vi "Main Page.vi"(8 "error in (no error)":errorcluster, 11 "Node Ptr":T2 format="%.0x") -> (0 "error out":errorcluster)   [LabVIEW 2020, in "SLSC-12201 DIO System Explorer.lvlib"]
uses:
  SLSC-12201 DIO System Explorer.lvlib
  <vilib>/NI VeriStand/Custom Device API/Custom Device Item Ref.ctl
  Direction Control.ctl
  Shared/Constants.vi
  <vilib>/NI VeriStand/Custom Device Tools/Custom Device Utility Library/NI VeriStand - Search for All Items by Name.vi
  <vilib>/NI VeriStand/Custom Device API/Get Item Property (Boolean).vi
  <vilib>/NI VeriStand/Custom Device Tools/Custom Device Utility Library/NI VeriStand - Search for Item by Name.vi
  <vilib>/NI VeriStand/Custom Device API/Get Item Property (I32).vi
  <vilib>/NI VeriStand/Custom Device API/Get Item Property (Variant).vi
  <vilib>/NI VeriStand/Custom Device API/Set Item Property (Variant).vi
  SLSC Pinout Window.vi
  SLSC Diagram Window.vi
  <vilib>/NI VeriStand/Custom Device API/Set Item Property (Boolean).vi
  <vilib>/NI VeriStand/Custom Device API/Set Item Property (String).vi
  <vilib>/NI VeriStand/Custom Device API/Custom Device API.lvlib
  Shared/SLSC-12201 DIO Shared.lvlib
  <vilib>/NI VeriStand/Custom Device Tools/Custom Device Utility Library/Custom Device Utility Library.lvlib
panel:
  in  "Loop rate":u32
  in  "rev A":bool
  in  "SHDocVw.IWebBrowser2":refnum<k7>(container)
  out "Version":string
  in  "Direction":T1 items=["Input", "Output Source", "Output Sink", "Output Push-Pull"]
  in  "Apply":bool
  in  "Enable":bool
  in  "Disable":bool
  in  "Tab Control":enum32{"Bank 0", "Bank 1"}(tab)
  in  "Input Threshold 5V Bank 0":dbl caption="Input Threshold"
  in  "Bank0 Select Vsup":u16(ring) caption="Voltage Supply" items=["Off", "Vsup_0", "Vsup_1"]
  in  "Pullup Resistor Bank 0":bool
  in  "Input Threshold 33V Bank 0":dbl caption="Input Threshold"
  in  "Enable 5V Range Bank 0":bool
  in  "Input Threshold 5V Bank 1":dbl caption="Input Threshold"
  in  "Bank1 Select Vsup":u16(ring) caption="Voltage Supply" items=["Off", "Vsup_0", "Vsup_1"]
  in  "Enable 5V Range Bank 1":bool
  in  "Pullup Resistor Bank 1":bool
  in  "Input Threshold 33V Bank 1":dbl caption="Input Threshold"
  in  "Tree":string[](tree)
  in  "Make Static Only":bool
  in  "Title":cluster{"Section Name":string}={"Section Name"="Custom Device Properties"}
  out "Module Number":i32
  in  "Header":cluster{"Section Name":string}={"Section Name"="Custom Device Item Settings"}
  in  "Description":string
  in  "Name":string
  # "ms"
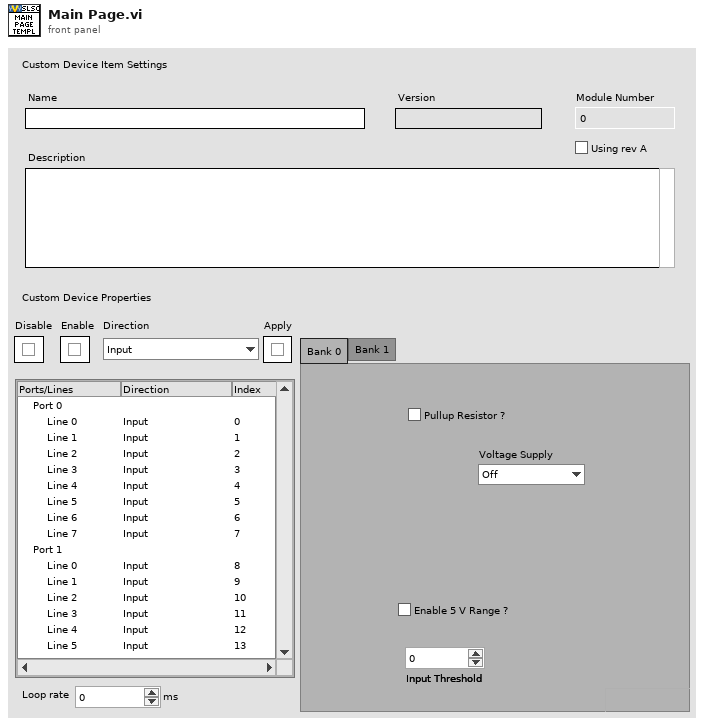
[diagram p1: front panel]
types:
  T1 = typedef "SLSC-12201 DIO System Explorer.lvlib/Direction Control.ctl" = u16
  T2 = typedef "Custom Device API.lvlib/Custom Device Item Ref.ctl" = u64
  T3 = enum8{"Enabled", "Disabled", "Disabled and Grayed Out"}
  T4 = typedef "Custom Device API.lvlib/Custom Device Channel.ctl" = cluster{"Type":T5, "Units":string, "Default Value":dbl, "Faultable":bool, "Scalable":bool}
  T5 = typedef "Custom Device API.lvlib/Custom Device Channel Type.ctl" = enum16{"Input", "Output"}
  T6 = cluster{"Channel Name":string, "SLSC Name":string, "Channel":T4, "Enum Names":string[], "Enum Values":i32[]}[]
  T7 = typedef "SLSC-12201 DIO System Explorer.lvlib/SLSC Channel Information.ctl" = cluster{"Channel Name":string, "SLSC Name":string, "Configuration":T4, "Enum Names":string[], "Enum Values":i32[]}
  T8 = typedef "Custom Device API.lvlib/Custom Device Item Info.ctl" = cluster{"Name":string, "Is Channel":bool, "GUID":string, "Is Waveform":bool}
  T9 = typedef "Custom Device API.lvlib/Custom Device Commands.ctl" = enum16{"Default", "Item renamed", "Shutdown", "Dynamic button pressed"}
  T10 = typedef "LVPoint32TypeDef.ctl" = cluster{"Horizontal":i32, "Vertical":i32}
  T11 = cluster{"Channel Name":string, "SLSC Name":string, "Channel":T4}[]
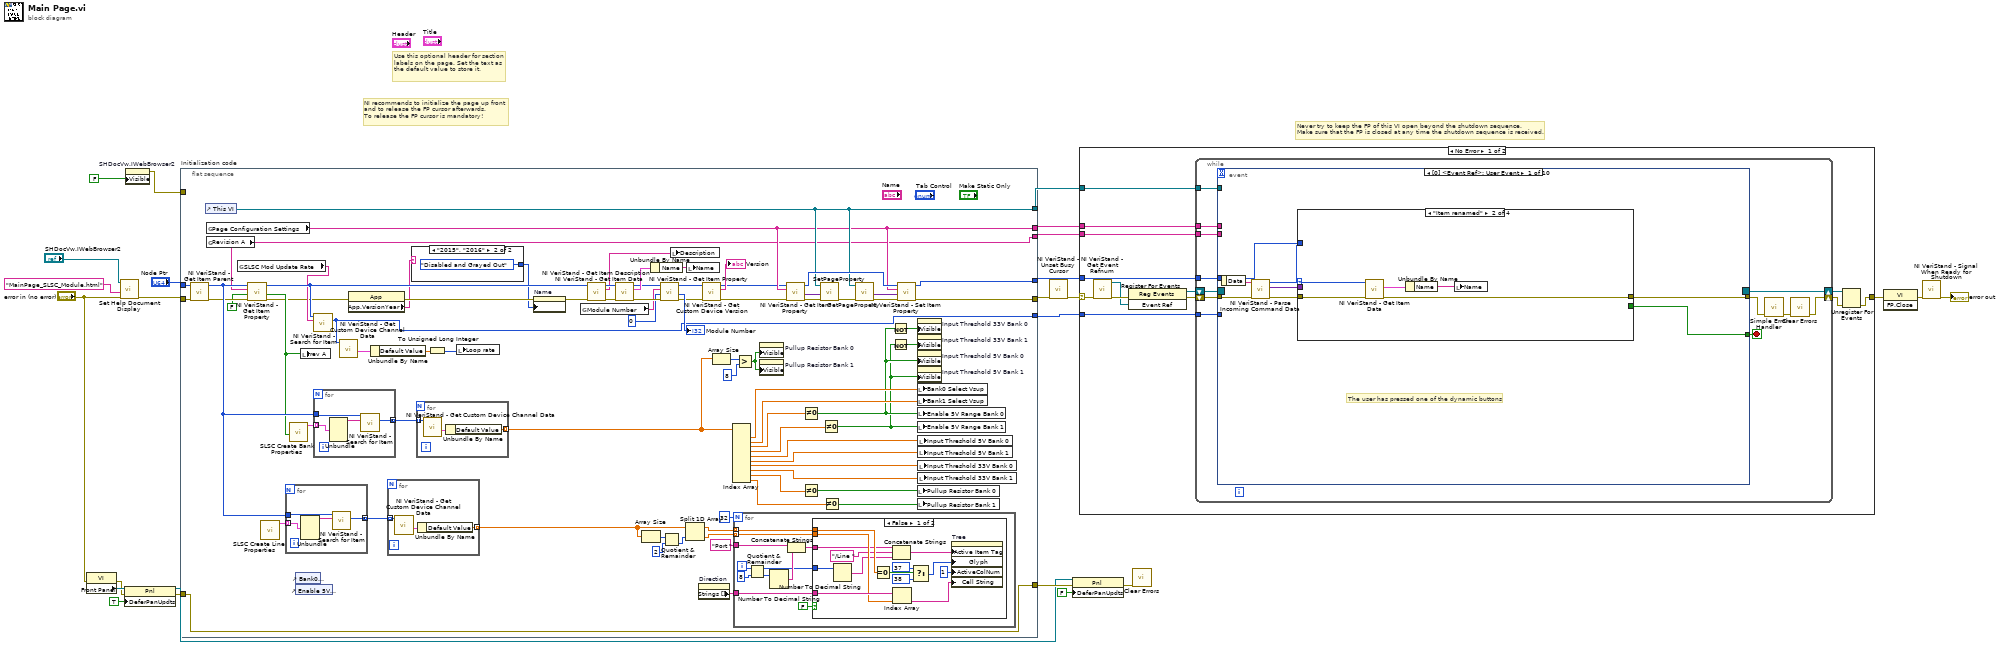
[diagram p0: block diagram]
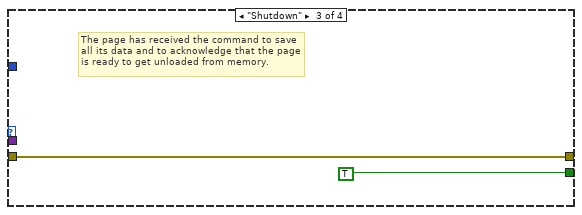
[diagram p3: hidden frame]
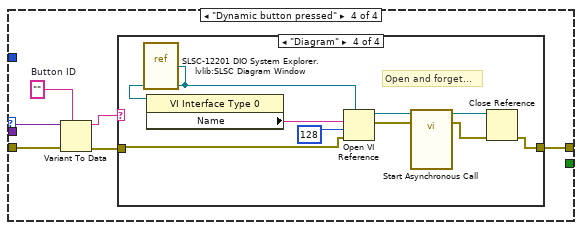
[diagram p4: hidden frame]
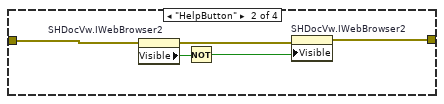
[diagram p6: hidden frame]
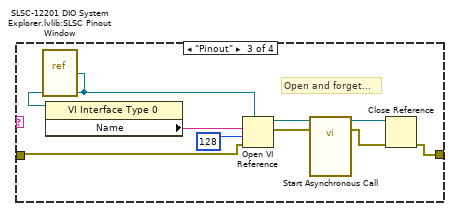
[diagram p7: hidden frame]
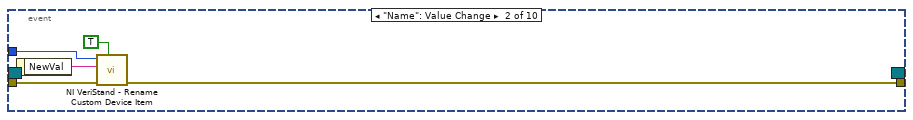
[diagram p8: hidden frame]
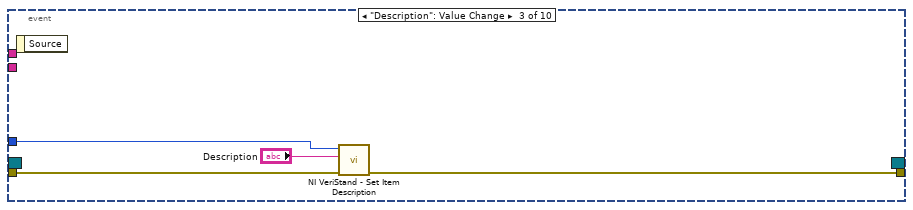
[diagram p9: hidden frame]
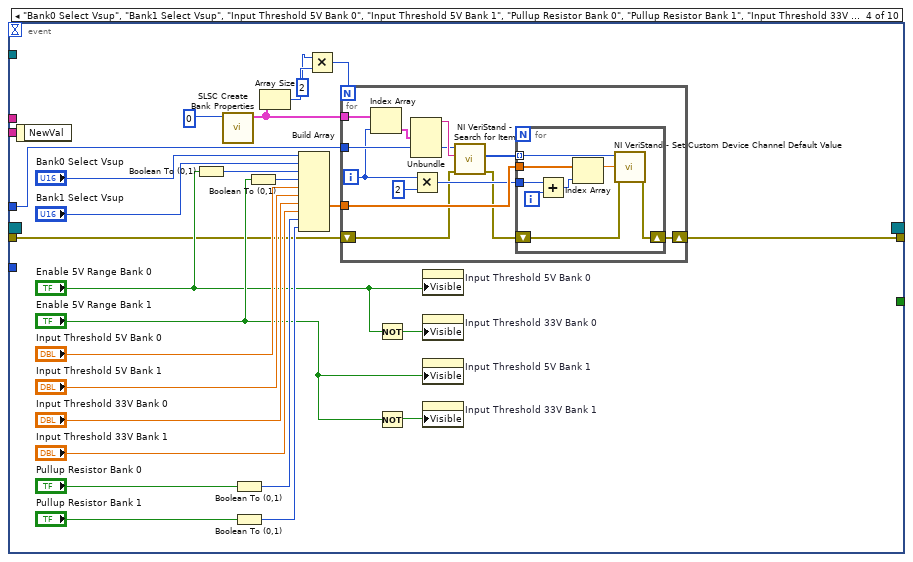
[diagram p10: hidden frame]
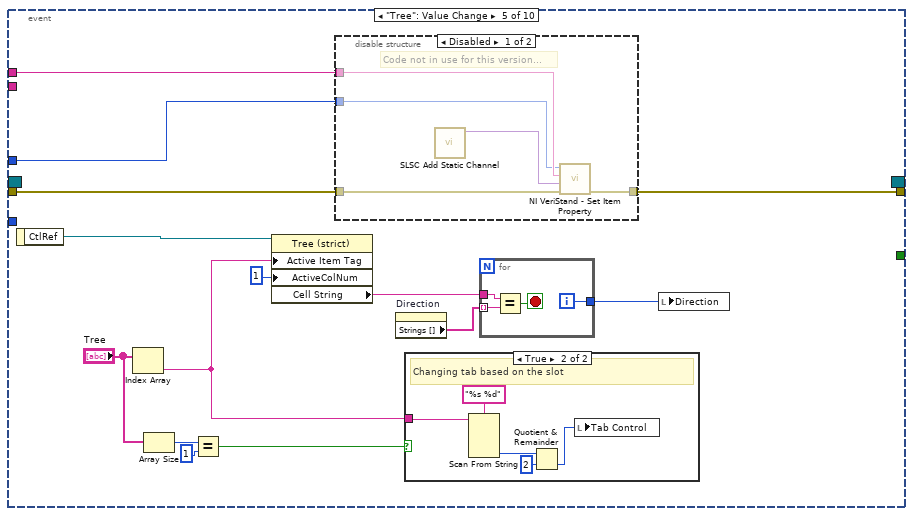
[diagram p11: hidden frame]
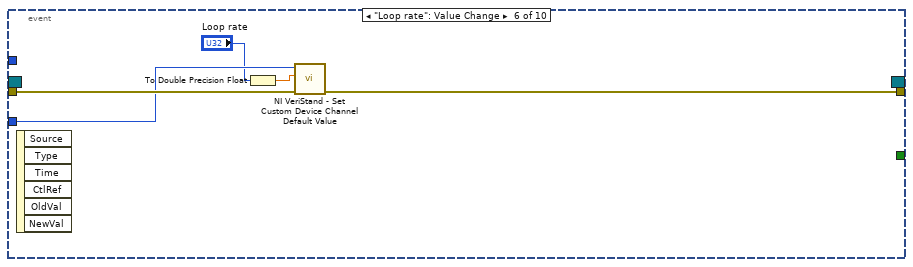
[diagram p14: hidden frame]
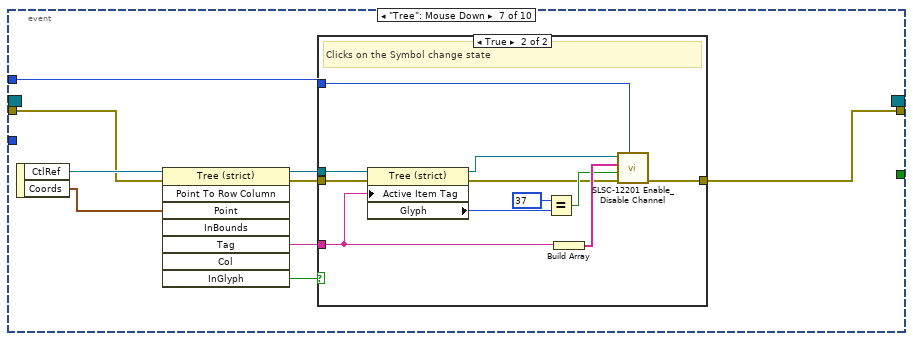
[diagram p15: hidden frame]
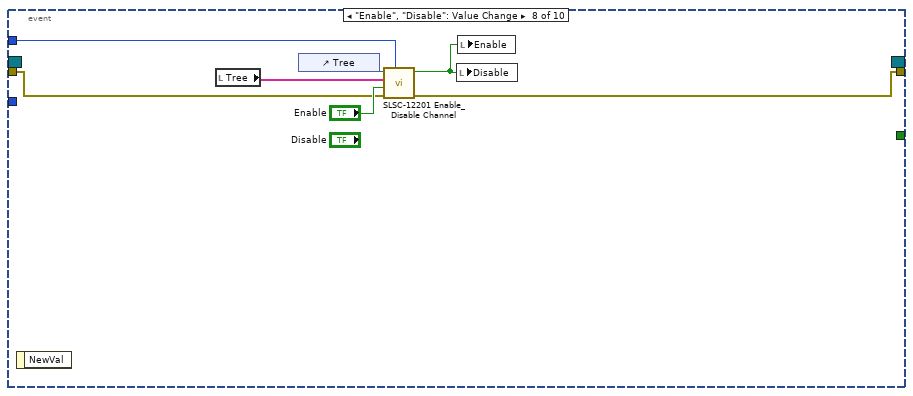
[diagram p17: hidden frame]
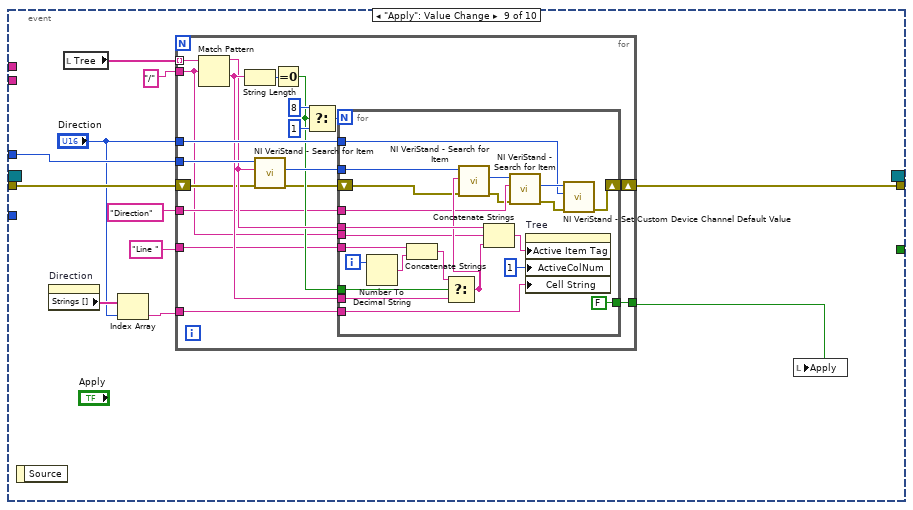
[diagram p18: hidden frame]
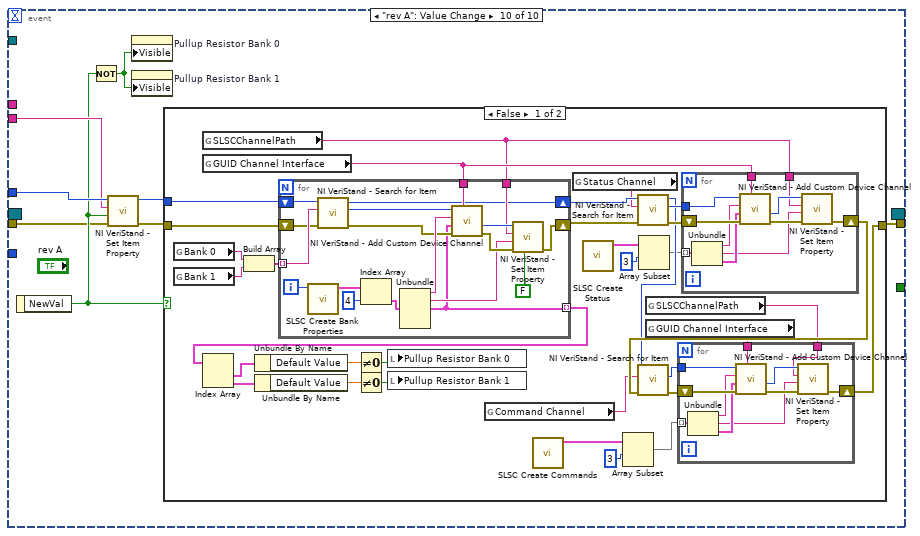
[diagram p19: hidden frame]
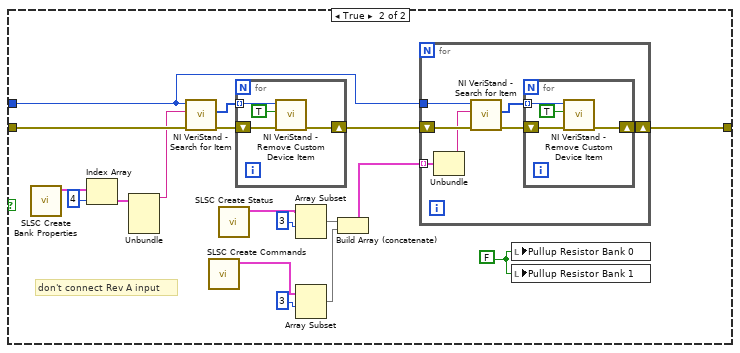
[diagram p20: hidden frame]
diagram:
  # "Never try to keep the FP of this VI open beyond the shutdown sequence.\nMake sure that the FP is closed at any time the shutdown sequence is received."
  # "Use this optional header for section labels on the page. Set the text as the default value to store it."
  # "NI recommends to initialize the page up front\nand to release the FP cursor afterwards.\nTo release the FP cursor is mandatory!"
  n1 = property class="VI"(error in="error in (no error)") -> (error out=w8:errorcluster, "Front Panel"=w10:refnum<vi>)  [unwired: 1 in, 1 out]
  n2 = call "Set Help Document Display.vi"("error in (no error)"="error in (no error)", "HTML File to Load"="MainPage_SLSC_Module.html" ("HTML File"), "SHDocVw.IWebBrowser2"="SHDocVw.IWebBrowser2") -> ("error out"=w13:errorcluster)  [unwired: 8 in]
  n3 = property class="Pnl"(reference=w10, error in=w8, "DeferPanUpdts"=TRUE ("Defer Panel Updates")) -> (reference out=w2:refnum<vi>, error out=w6:errorcluster)
  n4 = property on="SHDocVw.IWebBrowser2" class="AXCont"("Visible"=FALSE) -> (error out=w16:errorcluster)  [unwired: 2 in, 1 out]
  n5 = flat-sequence "Initialization code" {
    tunnel: w13 -> [w80]
    tunnel: "Node Ptr" -> [w81]
    tunnel: [w87] -> w21
    tunnel: [w84] -> w19
    tunnel: [w83] -> w18
    tunnel: [w82] -> w17
    tunnel: w16 -> [_]
    tunnel: [w38] -> w15
    tunnel: w6 -> [w36]
    tunnel: [w36] -> w4
    tunnel: [w30] -> w1
    frame #0 {
      n6 = call <vilib>:"NI VeriStand - Get Item Parent.vi"("error in (no error)"=w80, "Item Ref in"=w81) -> ("error out"=w40:errorcluster, "Item Ref out"=w41:T2)  [unwired: 6 in, 2 out]
      n7 = control-ref of="This VI"() -> (w83:refnum<vi>)
      n8 = global read "Constants.vi" "Page Configuration Settings"() -> (w82:string)
      n9 = global read "Constants.vi" "Revision A"() -> (w38:string)
      n10 = global read "Constants.vi" "SLSC Mod Update Rate"() -> (w31:string)
      n11 = call-poly <vilib>:"NI VeriStand - Get Item Property.vi"("error in (no error)"=w40, "Default Value"=FALSE, "Property Name"=w38, "Item Ref in"=w41) -> ("error out"=w29:errorcluster, "Value"=w37:bool, "Item Ref out"=w35:T2)  [unwired: 4 in, 1 out]
      n12 = call "SLSC Create Line Properties.vi"() -> ("Outgoing configuration"=w69:T6)  [unwired: 11 in]
      n13 = for {
        tunnel: w41 -> [w136]
        tunnel: w69 -> [w135] mode=indexing
        tunnel: [w134] -> w68 mode=concatenating
        n14 = Unbundle(w135) -> ("Channel Name"=w133:string)  [unwired: 4 out]
        n15 = call-poly <vilib>:"NI VeriStand - Search for Item.vi"("Item Name"=w133, "Section Ref in"=w136) -> ("Item Refs"=w134:T2[])  [unwired: 6 in, 3 out]
      }
      n16 = call "SLSC Create Bank Properties.vi"("RevA?"=w37) -> ("Outgoing configuration"=w76:T7[])  [unwired: 9 in, 1 out]
      n17 = control-ref of="Bank0 Select Vsup"() -> ()  [unwired: 1 out]
      n18 = control-ref of="Enable 5V Range Bank 0"() -> ()  [unwired: 1 out]
      n19 = local write "rev A"(w37) -> ()
      n20 = call-poly <vilib>:"NI VeriStand - Search for Item.vi"("Item Name"=w31, "Section Ref in"=w35) -> ("Item Ref"=w30:T2)  [unwired: 6 in, 3 out]
      n21 = for {
        tunnel: w41 -> [w140]
        tunnel: w76 -> [w138] mode=indexing
        tunnel: [w137] -> w75 mode=concatenating
        n22 = Unbundle(w138) -> ("Channel Name"=w139:string)  [unwired: 4 out]
        n23 = call-poly <vilib>:"NI VeriStand - Search for Item.vi"("Item Name"=w139, "Section Ref in"=w140) -> ("Item Refs"=w137:T2[])  [unwired: 6 in, 3 out]
      }
      n24 = call <vilib>:"NI VeriStand - Get Custom Device Channel Data.vi"("Channel Ref in"=w30) -> ("Channel"=w34:T4)  [unwired: 5 in, 5 out]
      n25 = property class="App"(error in=w29) -> (error out=w28:errorcluster, "App.VersionYear"=w27:string)  [unwired: 1 in, 1 out]
      n26 = Unbundle By Name(w34) -> ("Default Value"=w33:dbl)
      n27 = for {
        tunnel: [w132] -> w62 mode=indexing
        tunnel: w68 -> [w131] mode=indexing
        n28 = call <vilib>:"NI VeriStand - Get Custom Device Channel Data.vi"("Channel Ref in"=w131) -> ("Channel"=w130:T4)  [unwired: 5 in, 5 out]
        n29 = Unbundle By Name(w130) -> ("Default Value"=w132:dbl)
      }
      n30 = case shown="\"2015\", \"2016\"" w27 {
        tunnel: [T3."Enabled" ("Disabled") T3."Disabled and Grayed Out" ("Disabled")] -> w26
        frame "False", Default {
        }
        frame "2015", "2016" {
        }
      }
      n31 = for {
        tunnel: [w143] -> w54 mode=indexing
        tunnel: w75 -> [w142] mode=indexing
        n32 = call <vilib>:"NI VeriStand - Get Custom Device Channel Data.vi"("Channel Ref in"=w142) -> ("Channel"=w141:T4)  [unwired: 5 in, 5 out]
        n33 = Unbundle By Name(w141) -> ("Default Value"=w143:dbl)
      }
      n34 = To Unsigned Long Integer(number=w33) -> (unsigned 32bit integer=w32:u32)
      n35 = local write "Loop rate"(w32) -> ()
      n36 = property on="Name" class="Str"(error in=w28, "DisabledEnum"=w26) -> (error out=w97:errorcluster)  [unwired: 1 in, 1 out]
      n37 = global read "Constants.vi" "Module Number"() -> (w94:string)
      n38 = call <vilib>:"NI VeriStand - Get Item Description.vi"("error in (no error)"=w97, "Item Ref in"=w35) -> ("error out"=w100:errorcluster, "Description"=w101:string, "Item Ref out"=w102:T2)  [unwired: 7 out]
      n39 = call <vilib>:"NI VeriStand - Get Item Data.vi"("error in (no error)"=w100, "Item Ref in"=w102) -> ("error out"=w95:errorcluster, "Item Info"=w99:T8, "Item Ref out"=w93:T2)  [unwired: 7 out]
      n40 = Array Size(array=w62) -> (size(s)=w61:i32)
      n41 = Unbundle By Name(w99) -> ("Name"=w98:string)
      n42 = call-poly <vilib>:"NI VeriStand - Get Item Property.vi"("error in (no error)"=w95, "Default Value"=0, "Property Name"=w94, "Item Ref in"=w93) -> ("error out"=w45:errorcluster, "Value"=→"Module Number":i32, "Item Ref out"=w43:T2)  [unwired: 4 in, 1 out]
      n43 = Quotient & Remainder(x=w61, y=2) -> (floor(x/y)=w59:i32)  [unwired: 1 out]
      n44 = local write "Description"(w101) -> ()
      n45 = Split 1D Array(array=w62, index=w59) -> (first subarray=w67:dbl[], second subarray=w66:dbl[])
      n46 = local write "Name"(w98) -> ()
      n47 = property on="Direction" class="Ring (strict)"() -> ("Strings []"=w65:string[])  [unwired: 2 in, 2 out]
      n48 = call <vilib>:"NI VeriStand - Get Custom Device Version.vi"("error in (no error)"=w45, "Device Ref in"=w43) -> ("error out"=w44:errorcluster, "Value"=→"Version":string, "Device Ref out"=w42:T2)  [unwired: 7 in]
      n49 = Array Size(array=w54) -> (size(s)=w53:i32)
      n50 = Index Array(array=w54) -> (element #1=w79:dbl, element #2=w74:dbl, element #3=w73:dbl, element #4=w72:dbl, element #5=w58:dbl, element #6=w57:dbl, element #7=w56:dbl, element #8=w55:dbl, element #9=w71:dbl, element #10=w70:dbl)  [unwired: 10 in]
      n51 = for {
        N: 32 -> [_]
        tunnel: w67 -> [w115] mode=indexing
        tunnel: w66 -> [w113] mode=indexing
        tunnel: w65 -> [w114]
        tunnel: "Port " ("y") -> [w109]
        i -> [w112]
        n52 = Quotient & Remainder(x=w112, y=8) -> (x-y*floor(x/y)=w106:i32, floor(x/y)=w110:i32)
        n53 = Number To Decimal String(number=w110) -> (decimal integer string=w108:string)  [unwired: 1 in]
        n54 = Concatenate Strings(w109, w108) -> (w107:string)
        n55 = case shown="False" FALSE {
          tunnel: w115 -> [w125 _]
          tunnel: w114 -> [w123 _]
          tunnel: w113 -> [w122 _]
          tunnel: w107 -> [w118 _]
          tunnel: w106 -> [w116 _]
          frame False {
            n56 = Number To Decimal String(number=w116) -> (decimal integer string=w119:string)  [unwired: 1 in]
            n57 = Equal To 0?(x=w125) -> (x = 0?=w127:bool)
            n58 = Concatenate Strings(w118, "/Line " ("string"), w119) -> (w117:string)
            n59 = Index Array(array=w123, index=w122) -> (element=w121:string)
            n60 = Select(t=37, s=w127, f=38) -> (s? t:f=w126:i32)
            n61 = property on="Tree" class="Tree (strict)"("Active Item Tag"=w117, "Glyph"=w126, "ActiveColNum"=1 ("Active Cell:Active Column Number"), "Cell String"=w121) -> ()  [unwired: 2 in, 2 out]
          }
          frame True {
          }
        }
      }
      n62 = Greater?(x=w53, y=8) -> (0:w47:bool)
      n63 = property on="Pullup Resistor Bank 0" class="Bool (strict)"("Visible"=w47) -> ()  [unwired: 2 in, 2 out]
      n64 = property on="Pullup Resistor Bank 1" class="Bool (strict)"("Visible"=w47) -> ()  [unwired: 2 in, 2 out]
      n65 = call-poly <vilib>:"NI VeriStand - Get Item Property.vi"("error in (no error)"=w44, "Property Name"=w82, "Item Ref in"=w42) -> ("error out"=w91:errorcluster, "Value"=w90:variant, "Item Ref out"=w86:T2)  [unwired: 5 in, 1 out]
      n66 = Not Equal To 0?(x=w73) -> (x != 0?=w49:bool)
      n67 = Not Equal To 0?(x=w71) -> (x != 0?=w78:bool)
      n68 = call "SetPageProperty.vi"("error in"=w91, "variant"=w90, "This VI"=w83) -> ("error out"=w89:errorcluster)  [unwired: 8 in]
      n69 = Not Equal To 0?(x=w72) -> (x != 0?=w48:bool)
      n70 = Not Equal To 0?(x=w70) -> (x != 0?=w77:bool)
      n71 = call "GetPageProperty.vi"("error in (no error)"=w89, "This VI"=w83) -> ("error out"=w88:errorcluster, "Settings"=w85:variant)  [unwired: 8 in]
      n72 = Not(x=w49) -> (.not. x?=w51:bool)
      n73 = Not(x=w48) -> (.not. x?=w50:bool)
      n74 = call-poly <vilib>:"NI VeriStand - Set Item Property.vi"("error in (no error)"=w88, "Value"=w85, "Property Name"=w82, "Item Ref in"=w86) -> ("error out"=w87:errorcluster, "Item Ref out"=w84:T2)  [unwired: 5 in, 1 out]
      n75 = property on="Input Threshold 33V Bank 0" class="DigNum (strict)"("Visible"=w51) -> ()  [unwired: 2 in, 2 out]
      n76 = property on="Input Threshold 33V Bank 1" class="DigNum (strict)"("Visible"=w50) -> ()  [unwired: 2 in, 2 out]
      n77 = property on="Input Threshold 5V Bank 0" class="DigNum (strict)"("Visible"=w49) -> ()  [unwired: 2 in, 2 out]
      n78 = property on="Input Threshold 5V Bank 1" class="DigNum (strict)"("Visible"=w48) -> ()  [unwired: 2 in, 2 out]
      n79 = local write "Bank0 Select Vsup"(w79) -> ()
      n80 = local write "Bank1 Select Vsup"(w74) -> ()
      n81 = local write "Enable 5V Range Bank 0"(w49) -> ()
      n82 = local write "Enable 5V Range Bank 1"(w48) -> ()
      n83 = local write "Pullup Resistor Bank 0"(w78) -> ()
      n84 = local write "Pullup Resistor Bank 1"(w77) -> ()
      n85 = local write "Input Threshold 5V Bank 0"(w58) -> ()
      n86 = local write "Input Threshold 5V Bank 1"(w57) -> ()
      n87 = local write "Input Threshold 33V Bank 0"(w56) -> ()
      n88 = local write "Input Threshold 33V Bank 1"(w55) -> ()
    }
  }
  n89 = call <vilib>:"NI VeriStand - Unset Busy Cursor.vi"("error in (no error)"=w21) -> ("error out"=w20:errorcluster)  [unwired: 10 out]
  n90 = property class="Pnl"(reference=w2, error in=w4, "DeferPanUpdts"=FALSE ("Defer Panel Updates")) -> (error out=w3:errorcluster)  [unwired: 1 out]
  n91 = case shown="No Error" w20 {
    selector: w20 -> [w148 w500]
    tunnel: [w153 w498] -> w25
    tunnel: w19 -> [w149 _]
    tunnel: w18 -> [w147 _]
    tunnel: w17 -> [w146 _]
    tunnel: w15 -> [w145 _]
    tunnel: w1 -> [w144 _]
    frame No Error {
      n92 = call <vilib>:"NI VeriStand - Get Event Refnum.vi"("error in (no error)"=w148) -> ("error out"=w156:errorcluster, "Event Ref"=w152:refnum<user-event>)  [unwired: 9 out]
      n93 = register-events(error in=w156, w152) -> (reference out=w150:refnum<event-registration>, error out=w151:errorcluster)  [unwired: 1 in]
      n94 = while {
        tunnel: w149 -> [w164]
        shift-right: [w161] -> w154
        shift-left: w151 -> [w167]
        shift-right: [w168] -> w155
        shift-left: w150 -> [w166]
        tunnel: w147 -> [w160]
        tunnel: w146 -> [w159]
        tunnel: w145 -> [w158]
        tunnel: w144 -> [w157]
        stop <- w165 stop-if-true
        n95 = event shown="[0] <Event Ref>: User Event" {
          selector: w166 -> [_ _ _ _ _ _ _ _ _ _]
          dyn-events: [_ _ _ _ _ _ _ _ _ _] -> w168
          timeout: _ -> [_ _ _ _ _ _ _ _ _ _]
          tunnel: w167 -> [w176 w218 w222 w225 w281 w301 w309 w326 w335 w384]
          tunnel: [w172 _ _ _ _ _ _ _ _ _] -> w165
          tunnel: [w171 w217 w221 w224 w282 w300 w305 w325 w334 w390] -> w163
          tunnel: w164 -> [w170 w219 w223 w247 w279 _ w306 w329 w340 w388]
          tunnel: w160 -> [_ _ _ _ _ _ _ _ _ _]
          tunnel: w159 -> [_ _ _ _ w280 _ _ _ _ _]
          tunnel: w158 -> [_ _ _ _ _ _ _ _ _ w386]
          tunnel: w157 -> [_ _ _ _ _ w299 _ _ _ _]
          event User Event {
            # "The user has pressed one of the dynamic buttons"
            n96 = event-data() -> ("Data"=w175:string)  [unwired: 1 out]
            n97 = call <vilib>:"NI VeriStand - Parse Incoming Command Data.vi"("error in (no error)"=w176, "Incoming data"=w175) -> ("error out"=w174:errorcluster, "Outgoing data"=w169:variant, "Action"=w173:T9)  [unwired: 7 out]
            n98 = case shown="\"Item renamed\"" w173 {
              tunnel: w174 -> [w177 w182 w183 w190]
              tunnel: [_ _ TRUE _] -> w172
              tunnel: [w177 w179 w183 w185] -> w171
              tunnel: w170 -> [_ w181 _ _]
              tunnel: w169 -> [_ _ _ w189]
              frame "Default", Default {
              }
              frame "Item renamed" {
                n99 = call <vilib>:"NI VeriStand - Get Item Data.vi"("error in (no error)"=w182, "Item Ref in"=w181) -> ("error out"=w179:errorcluster, "Item Info"=w180:T8)  [unwired: 8 out]
                n100 = Unbundle By Name(w180) -> ("Name"=w178:string)
                n101 = local write "Name"(w178) -> ()
              }
              frame "Shutdown" {
                # "The page has received the command to save all its data and to acknowledge that the page is ready to get unloaded from memory."
              }
              frame "Dynamic button pressed" {
                w188 = ""  # Button ID
                n102 = Variant To Data(error in=w190, type=w188, Variant=w189) -> (data=w187:string, error out=w186:errorcluster)
                n103 = case shown="\"Diagram\"" w187 {
                  tunnel: w186 -> [w191 w194 w198 w207]
                  tunnel: [w191 w192 w199 w208] -> w185
                  frame Default {
                  }
                  frame "HelpButton" {
                    n104 = property on="SHDocVw.IWebBrowser2" class="AXCont"(error in=w194) -> (error out=w193:errorcluster, "Visible"=w196:bool)  [unwired: 1 in, 1 out]
                    n105 = Not(x=w196) -> (.not. x?=w195:bool)
                    n106 = property on="SHDocVw.IWebBrowser2" class="AXCont"(error in=w193, "Visible"=w195) -> (error out=w192:errorcluster)  [unwired: 1 in, 1 out]
                  }
                  frame "Pinout" {
                    # "Open and forget..."
                    n107 = vi-ref "SLSC-12201 DIO System Explorer.lvlib:SLSC Pinout Window.vi"() -> (w197:refnum<vi>)
                    n108 = property class="VI Interface Type 0"(reference=w197) -> ("Name"=w205:string)  [unwired: 1 in, 2 out]
                    n109 = Open VI Reference(type specifier VI Refnum (for type only)=w197, vi path=w205, options=128, error in (no error)=w198) -> (vi reference=w201:refnum<vi>, error out=w203:errorcluster)  [unwired: 2 in]
                    n110 = call-by-ref "Start Asynchronous Call"(reference=w201, error in=w203) -> (reference out=w202:refnum<vi>, error out=w204:errorcluster)  [unwired: 12 in]
                    n111 = Close Reference(reference=w202, error in (no error)=w204) -> (error out=w199:errorcluster)
                  }
                  frame "Diagram" {
                    # "Open and forget..."
                    n112 = vi-ref "SLSC-12201 DIO System Explorer.lvlib:SLSC Diagram Window.vi"() -> (w206:refnum<vi>)
                    n113 = property class="VI Interface Type 0"(reference=w206) -> ("Name"=w214:string)  [unwired: 1 in, 2 out]
                    n114 = Open VI Reference(type specifier VI Refnum (for type only)=w206, vi path=w214, options=128, error in (no error)=w207) -> (vi reference=w210:refnum<vi>, error out=w212:errorcluster)  [unwired: 2 in]
                    n115 = call-by-ref "Start Asynchronous Call"(reference=w210, error in=w212) -> (reference out=w211:refnum<vi>, error out=w213:errorcluster)  [unwired: 12 in]
                    n116 = Close Reference(reference=w211, error in (no error)=w213) -> (error out=w208:errorcluster)
                  }
                }
              }
            }
          }
          event "Name": Value Change {
            n117 = event-data() -> ("NewVal"=w216:string)  [unwired: 1 out]
            n118 = call <vilib>:"NI VeriStand - Rename Custom Device Item.vi"("Force Rename (F)"=TRUE, "error in (no error)"=w218, "New Name"=w216, "Item Ref in"=w219) -> ("error out"=w217:errorcluster)  [unwired: 7 out]
          }
          event "Description": Value Change {
            n119 = event-data() -> ()  [unwired: 2 out]
            n120 = call <vilib>:"NI VeriStand - Set Item Description.vi"("error in (no error)"=w222, "Description"="Description", "Item Ref in"=w223) -> ("error out"=w221:errorcluster)  [unwired: 8 out]
          }
          event "Bank0 Select Vsup", "Bank1 Select Vsup", "Input Threshold 5V Bank 0", "Input Threshold 5V Bank 1", "Pullup Resistor Bank 0", "Pullup Resistor Bank 1", "Input Threshold 33V Bank 0", "Input Threshold 33V Bank 1", "Enable 5V Range Bank 1", "Enable 5V Range Bank 0": Value Change {
            n121 = event-data() -> ()  [unwired: 2 out]
            n122 = Boolean To (0,1)(Boolean="Enable 5V Range Bank 0") -> (0, 1=w243:i16)
            n123 = call "SLSC Create Bank Properties.vi"("Bank Number"=0) -> ("Outgoing configuration"=w233:T7[])  [unwired: 9 in, 1 out]
            n124 = Boolean To (0,1)(Boolean="Pullup Resistor Bank 0") -> (0, 1=w235:i16)
            n125 = Boolean To (0,1)(Boolean="Pullup Resistor Bank 1") -> (0, 1=w234:i16)
            n126 = Boolean To (0,1)(Boolean="Enable 5V Range Bank 1") -> (0, 1=w242:i16)
            n127 = Array Size(array=w233) -> (size(s)=w231:i32)
            n128 = Build Array("Bank0 Select Vsup", "Bank1 Select Vsup", w243, w242, "Input Threshold 5V Bank 0", "Input Threshold 5V Bank 1", "Input Threshold 33V Bank 0", "Input Threshold 33V Bank 1", w235, w234) -> (w244:dbl[])
            n129 = Multiply(x=2 ("y"), y=w231) -> (x*y=w232:i32)
            n130 = for {
              N: w232 -> [_]
              tunnel: w247 -> [w259]
              tunnel: w244 -> [w257]
              tunnel: w233 -> [w256]
              shift-right: [w249] -> w224
              shift-left: w225 -> [w251]
              i -> [w253]
              n131 = Index Array(array=w256, index=w253) -> (element=w255:T7)
              n132 = Unbundle(w255) -> ("Channel Name"=w260:string)  [unwired: 4 out]
              n133 = Multiply(x=w253, y=2) -> (x*y=w252:i32)
              n134 = call-poly <vilib>:"NI VeriStand - Search for Item.vi"("error in"=w251, "Item Name"=w260, "Section Ref in"=w259) -> ("error out"=w250:errorcluster, "Item Refs"=w258:T2[])  [unwired: 5 in, 2 out]
              n135 = for {
                tunnel: w257 -> [w268]
                tunnel: w258 -> [w267] mode=indexing
                tunnel: w252 -> [w263]
                shift-right: [w261] -> w249
                shift-left: w250 -> [w262]
                i -> [w265]
                n136 = Add(x=w263, y=w265) -> (x+y=w264:i32)
                n137 = Index Array(array=w268, index=w264) -> (element=w266:dbl)
                n138 = call <vilib>:"NI VeriStand - Set Custom Device Channel Default Value.vi"("error in (no error)"=w262, "Default Value"=w266, "Channel Ref in"=w267) -> ("error out"=w261:errorcluster)  [unwired: 7 in, 1 out]
              }
            }
            n139 = Not(x="Enable 5V Range Bank 0") -> (.not. x?=w229:bool)
            n140 = Not(x="Enable 5V Range Bank 1") -> (.not. x?=w228:bool)
            n141 = property on="Input Threshold 5V Bank 0" class="DigNum (strict)"("Visible"="Enable 5V Range Bank 0") -> ()  [unwired: 2 in, 2 out]
            n142 = property on="Input Threshold 33V Bank 0" class="DigNum (strict)"("Visible"=w229) -> ()  [unwired: 2 in, 2 out]
            n143 = property on="Input Threshold 5V Bank 1" class="DigNum (strict)"("Visible"="Enable 5V Range Bank 1") -> ()  [unwired: 2 in, 2 out]
            n144 = property on="Input Threshold 33V Bank 1" class="DigNum (strict)"("Visible"=w228) -> ()  [unwired: 2 in, 2 out]
          }
          event "Tree": Value Change {
            n145 = event-data() -> ("CtlRef"=w278:refnum<vi>)  [unwired: 1 out]
            n146 = Index Array(array="Tree") -> (element=w269:string)  [unwired: 1 in]
            n147 = Array Size(array="Tree") -> (size(s)=w272:i32)
            n148 = Equal?(x=w272, y=1) -> (x = y?=w270:bool)
            n149 = property on="Property Node" class="Tree (strict)"(reference=w278, "Active Item Tag"=w269, "ActiveColNum"=1 ("Active Cell:Active Column Number")) -> ("Cell String"=w275:string)  [unwired: 1 in, 2 out]
            n150 = disable-structure shown="Disabled" {
              disable-tunnel: [w296 w297] -> w282
              disable-tunnel: w281 -> [w295 w297]
              disable-tunnel: w280 -> [w293 _]
              disable-tunnel: w279 -> [w292 _]
              frame Disabled {
                # "Code not in use for this version..."
                n151 = call "SLSC Add Static Channel.vi"() -> ("variant out"=w294:variant)  [unwired: 10 in, 1 out]
                n152 = call-poly <vilib>:"NI VeriStand - Set Item Property.vi"("error in (no error)"=w295, "Value"=w294, "Property Name"=w293, "Item Ref in"=w292) -> ("error out"=w296:errorcluster)  [unwired: 5 in, 2 out]
              }
              frame Enabled {
              }
            }
            n153 = property on="Direction" class="Ring (strict)"() -> ("Strings []"=w276:string[])  [unwired: 2 in, 2 out]
            n154 = case shown="True" w270 {
              tunnel: w269 -> [_ w286]
              frame False {
              }
              frame True {
                # "Changing tab based on the slot"
                n155 = Scan From String(format string="%s %d", input string=w286) -> (output 2=w285:i32)  [unwired: 5 in, 3 out]
                n156 = Quotient & Remainder(x=w285, y=2) -> (floor(x/y)=w283:i32)  [unwired: 1 out]
                n157 = local write "Tab Control"(w283) -> ()
              }
            }
            n158 = for {
              tunnel: w276 -> [w291] mode=indexing
              tunnel: w275 -> [w290]
              tunnel: [w288] -> w274
              i -> [w288]
              stop <- w289 stop-if-true
              n159 = Equal?(x=w290, y=w291) -> (x = y?=w289:bool)
            }
            n160 = local write "Direction"(w274) -> ()
          }
          event "Loop rate": Value Change {
            n161 = event-data() -> ()  [unwired: 7 out]
            n162 = To Double Precision Float(number="Loop rate") -> (double precision float=w302:dbl)
            n163 = call <vilib>:"NI VeriStand - Set Custom Device Channel Default Value.vi"("error in (no error)"=w301, "Default Value"=w302, "Channel Ref in"=w299) -> ("error out"=w300:errorcluster)  [unwired: 7 in, 1 out]
          }
          event "Tree": Mouse Down {
            n164 = event-data() -> ("CtlRef"=w311:refnum<vi>, "Coords"=w310:T10)  [unwired: 1 out]
            n165 = invoke class="Tree (strict)" method="Point To Row Column"(reference=w311, error in=w309, "Point"=w310) -> (reference out=w304:refnum<vi>, error out=w303:errorcluster, "Tag"=w307:string, "InGlyph"=w308:bool)  [unwired: 5 in, 4 out]
            n166 = case shown="True" w308 {
              tunnel: w307 -> [_ w318]
              tunnel: w306 -> [_ w322]
              tunnel: [w312 w321] -> w305
              tunnel: w304 -> [_ w320]
              tunnel: w303 -> [w312 w314]
              frame False {
              }
              frame True {
                # "Clicks on the Symbol change state"
                n167 = property on="Property Node" class="Tree (strict)"(reference=w320, error in=w314, "Active Item Tag"=w318) -> (reference out=w319:refnum<vi>, error out=w313:errorcluster, "Glyph"=w317:i32)
                n168 = Equal?(x=37, y=w317) -> (x = y?=w315:bool)
                n169 = Build Array(w318) -> (w323:string[])
                n170 = call "SLSC-12201 Enable_Disable Channel.vi"("Item Ref in"=w322, "error in (no error)"=w313, "Enable"=w315, "Tree"=w323, "TreeControl in"=w319) -> ("error out"=w321:errorcluster)  [unwired: 5 in, 1 out]
              }
            }
          }
          event "Enable", "Disable": Value Change {
            n171 = event-data() -> ()  [unwired: 2 out]
            n172 = local read "Tree"() -> (w330:string[])
            n173 = control-ref of="Tree"() -> (w324:refnum<vi>)
            n174 = call "SLSC-12201 Enable_Disable Channel.vi"("Item Ref in"=w329, "error in (no error)"=w326, "Enable"="Enable", "Tree"=w330, "TreeControl in"=w324) -> ("error out"=w325:errorcluster, "Boolean"=w327:bool)  [unwired: 5 in]
            n175 = local write "Disable"(w327) -> ()
            n176 = local write "Enable"(w327) -> ()
          }
          event "Apply": Value Change {
            n177 = event-data() -> ()  [unwired: 2 out]
            n178 = property on="Direction" class="Ring (strict)"() -> ("Strings []"=w333:string[])  [unwired: 2 in, 2 out]
            n179 = local read "Tree"() -> (w341:string[])
            n180 = Index Array(array=w333, index="Direction") -> (element=w331:string)
            n181 = for {
              tunnel: w341 -> [w354] mode=indexing
              tunnel: w331 -> [w356]
              tunnel: w340 -> [w355]
              tunnel: "Direction" -> [w352]
              tunnel: [w350] -> w339
              tunnel: "/" ("regular expression") -> [w342]
              tunnel: "Line " ("string") -> [w347]
              tunnel: "Direction" ("Item Name") -> [w346]
              shift-right: [w343] -> w334
              shift-left: w335 -> [w345]
              n182 = Match Pattern(string=w354, regular expression=w342) -> (before substring=w349:string, after substring=w351:string)  [unwired: 1 in, 2 out]
              n183 = String Length(string=w351) -> (length=w360:i32)
              n184 = call-poly <vilib>:"NI VeriStand - Search for Item.vi"("error in"=w345, "Item Name"=w349, "Section Ref in"=w355) -> ("error out"=w344:errorcluster, "Item Ref"=w353:T2)  [unwired: 5 in, 2 out]
              n185 = Equal To 0?(x=w360) -> (x = 0?=w348:bool)
              n186 = Select(t=8, s=w348, f=1) -> (s? t:f=w359:i32)
              n187 = for {
                N: w359 -> [_]
                tunnel: w349 -> [w379]
                tunnel: w356 -> [w361]
                tunnel: w353 -> [w380]
                tunnel: w352 -> [w362]
                tunnel: w348 -> [w376]
                tunnel: w351 -> [w373]
                tunnel: [FALSE] -> w350
                tunnel: w347 -> [w371]
                tunnel: w346 -> [w370]
                shift-right: [w366] -> w343
                shift-left: w344 -> [w369]
                tunnel: w342 -> [w365]
                i -> [w382]
                n188 = Number To Decimal String(number=w382) -> (decimal integer string=w381:string)  [unwired: 1 in]
                n189 = Concatenate Strings(w371, w381) -> (w375:string)
                n190 = Select(t=w375, s=w376, f=w373) -> (s? t:f=w374:string)
                n191 = call-poly <vilib>:"NI VeriStand - Search for Item.vi"("error in"=w369, "Item Name"=w374, "Section Ref in"=w380) -> ("error out"=w368:errorcluster, "Item Ref"=w378:T2)  [unwired: 5 in, 2 out]
                n192 = Concatenate Strings(w379, w365, w374) -> (w364:string)
                n193 = call-poly <vilib>:"NI VeriStand - Search for Item.vi"("error in"=w368, "Item Name"=w370, "Section Ref in"=w378) -> ("error out"=w367:errorcluster, "Item Ref"=w377:T2)  [unwired: 5 in, 2 out]
                n194 = property on="Tree" class="Tree (strict)"("Active Item Tag"=w364, "ActiveColNum"=1 ("Active Cell:Active Column Number"), "Cell String"=w361) -> ()  [unwired: 2 in, 2 out]
                n195 = call <vilib>:"NI VeriStand - Set Custom Device Channel Default Value.vi"("error in (no error)"=w367, "Default Value"=w362, "Channel Ref in"=w377) -> ("error out"=w366:errorcluster)  [unwired: 7 in, 1 out]
              }
            }
            n196 = local write "Apply"(w339) -> ()
          }
          event "rev A": Value Change {
            n197 = event-data() -> ("NewVal"=w385:bool)  [unwired: 1 out]
            n198 = Not(x=w385) -> (.not. x?=w389:bool)
            n199 = call-poly <vilib>:"NI VeriStand - Set Item Property.vi"("error in (no error)"=w384, "Value"=w385, "Property Name"=w386, "Item Ref in"=w388) -> ("error out"=w383:errorcluster, "Item Ref out"=w387:T2)  [unwired: 5 in, 1 out]
            n200 = property on="Pullup Resistor Bank 0" class="Bool (strict)"("Visible"=w389) -> ()  [unwired: 2 in, 2 out]
            n201 = property on="Pullup Resistor Bank 1" class="Bool (strict)"("Visible"=w389) -> ()  [unwired: 2 in, 2 out]
            n202 = case shown="False" w385 {
              tunnel: w387 -> [w423 w471]
              tunnel: w383 -> [w419 w482]
              tunnel: [w403 w474] -> w390
              frame False {
                n203 = global read "Constants.vi" "Bank 0"() -> (w421:string)
                n204 = global read "Constants.vi" "Bank 1"() -> (w422:string)
                n205 = global read "Constants.vi" "SLSCChannelPath"() -> (w400:string)
                n206 = global read "Constants.vi" "GUID Channel Interface"() -> (w401:string)
                n207 = Build Array(w421, w422) -> (w420:string[])
                n208 = for {
                  tunnel: w420 -> [w463] mode=indexing
                  shift-right: [w451] -> w408
                  shift-left: w419 -> [w452]
                  tunnel: [w450] -> w418 mode=indexing
                  tunnel: w400 -> [w449]
                  tunnel: w401 -> [w448]
                  shift-right: [w446] -> w410
                  shift-left: w423 -> [w464]
                  i -> [w459]
                  n209 = call "SLSC Create Bank Properties.vi"("Bank Number"=w459) -> ("Outgoing configuration"=w458:T7[])  [unwired: 9 in, 1 out]
                  n210 = call-poly <vilib>:"NI VeriStand - Search for Item.vi"("error in"=w452, "Item Name"=w463, "Section Ref in"=w464) -> ("error out"=w453:errorcluster, "Item Ref"=w460:T2, "Section Ref out"=w446:T2)  [unwired: 5 in, 1 out]
                  n211 = Index Array(array=w458, index=4) -> (element=w456:T7)
                  n212 = Unbundle(w456) -> ("Channel Name"=w455:string, "SLSC Name"=w454:string, "Configuration"=w450:T4)  [unwired: 2 out]
                  n213 = call <vilib>:"NI VeriStand - Add Custom Device Channel.vi"("GUID (Default Channel)"=w448, "error in (no error)"=w453, "Channel"=w450, "Channel Name"=w455, "Parent Ref in"=w460) -> ("error out"=w461:errorcluster, "Channel Ref"=w462:T2)  [unwired: 3 in, 2 out]
                  n214 = call-poly <vilib>:"NI VeriStand - Set Item Property.vi"("Binary String (T)"=FALSE, "error in (no error)"=w461, "Value"=w454, "Property Name"=w449, "Item Ref in"=w462) -> ("error out"=w451:errorcluster)  [unwired: 4 in, 2 out]
                }
                n215 = Index Array(array=w418) -> (element #1=w417:T4, element #2=w416:T4)  [unwired: 2 in]
                n216 = Unbundle By Name(w417) -> ("Default Value"=w415:dbl)
                n217 = Unbundle By Name(w416) -> ("Default Value"=w413:dbl)
                n218 = Not Equal To 0?(x=w415) -> (x != 0?=w414:bool)
                n219 = Not Equal To 0?(x=w413) -> (x != 0?=w412:bool)
                n220 = local write "Pullup Resistor Bank 0"(w414) -> ()
                n221 = local write "Pullup Resistor Bank 1"(w412) -> ()
                n222 = global read "Constants.vi" "Command Channel"() -> (w399:string)
                n223 = call "SLSC Create Commands.vi"() -> ("Outgoing configuration"=w392:T11)  [unwired: 11 in]
                n224 = global read "Constants.vi" "Status Channel"() -> (w409:string)
                n225 = call "SLSC Create Status.vi"() -> ("Outgoing configuration"=w395:T11)  [unwired: 11 in]
                n226 = Array Subset(array=w392, index=3) -> (w391:T11)  [unwired: 1 in]
                n227 = call-poly <vilib>:"NI VeriStand - Search for Item.vi"("error in"=w408, "Item Name"=w409, "Section Ref in"=w410) -> ("error out"=w411:errorcluster, "Item Ref"=w407:T2, "Section Ref out"=w402:T2)  [unwired: 5 in, 1 out]
                n228 = Array Subset(array=w395, index=3) -> (w394:T11)  [unwired: 1 in]
                n229 = global read "Constants.vi" "SLSCChannelPath"() -> (w398:string)
                n230 = global read "Constants.vi" "GUID Channel Interface"() -> (w397:string)
                n231 = for {
                  tunnel: w407 -> [w441]
                  shift-right: [w435] -> w404
                  shift-left: w411 -> [w440]
                  tunnel: w400 -> [w443]
                  tunnel: w401 -> [w442]
                  tunnel: w394 -> [w439] mode=indexing
                  n232 = Unbundle(w439) -> ("Channel Name"=w438:string, "SLSC Name"=w436:string, "Channel"=w437:T4)
                  n233 = call <vilib>:"NI VeriStand - Add Custom Device Channel.vi"("GUID (Default Channel)"=w442, "error in (no error)"=w440, "Channel"=w437, "Channel Name"=w438, "Parent Ref in"=w441) -> ("error out"=w444:errorcluster, "Channel Ref"=w445:T2)  [unwired: 3 in, 2 out]
                  n234 = call-poly <vilib>:"NI VeriStand - Set Item Property.vi"("error in (no error)"=w444, "Value"=w436, "Property Name"=w443, "Item Ref in"=w445) -> ("error out"=w435:errorcluster)  [unwired: 5 in, 2 out]
                }
                n235 = call-poly <vilib>:"NI VeriStand - Search for Item.vi"("error in"=w404, "Item Name"=w399, "Section Ref in"=w402) -> ("error out"=w405:errorcluster, "Item Ref"=w406:T2)  [unwired: 5 in, 2 out]
                n236 = for {
                  tunnel: w406 -> [w429]
                  shift-right: [w432] -> w403
                  shift-left: w405 -> [w428]
                  tunnel: w398 -> [w431]
                  tunnel: w397 -> [w430]
                  tunnel: w391 -> [w427] mode=indexing
                  n237 = Unbundle(w427) -> ("Channel Name"=w426:string, "SLSC Name"=w424:string, "Channel"=w425:T4)
                  n238 = call <vilib>:"NI VeriStand - Add Custom Device Channel.vi"("GUID (Default Channel)"=w430, "error in (no error)"=w428, "Channel"=w425, "Channel Name"=w426, "Parent Ref in"=w429) -> ("error out"=w433:errorcluster, "Channel Ref"=w434:T2)  [unwired: 3 in, 2 out]
                  n239 = call-poly <vilib>:"NI VeriStand - Set Item Property.vi"("error in (no error)"=w433, "Value"=w424, "Property Name"=w431, "Item Ref in"=w434) -> ("error out"=w432:errorcluster)  [unwired: 5 in, 2 out]
                }
              }
              frame True {
                w475 = FALSE ("Pullup Resistor Bank 0")
                # "don't connect Rev A input"
                n240 = call "SLSC Create Bank Properties.vi"() -> ("Outgoing configuration"=w479:T7[])  [unwired: 10 in, 1 out]
                n241 = Index Array(array=w479, index=4) -> (element=w477:T7)
                n242 = Unbundle(w477) -> ("Channel Name"=w476:string)  [unwired: 4 out]
                n243 = call-poly <vilib>:"NI VeriStand - Search for Item.vi"("error in"=w482, "Item Name"=w476, "Section Ref in"=w471) -> ("error out"=w480:errorcluster, "Item Refs"=w481:T2[])  [unwired: 5 in, 2 out]
                n244 = call "SLSC Create Commands.vi"() -> ("Outgoing configuration"=w467:T11)  [unwired: 11 in]
                n245 = call "SLSC Create Status.vi"() -> ("Outgoing configuration"=w472:T11)  [unwired: 11 in]
                n246 = for {
                  tunnel: w481 -> [w497] mode=indexing
                  shift-right: [w495] -> w470
                  shift-left: w480 -> [w496]
                  n247 = call <vilib>:"NI VeriStand - Remove Custom Device Item.vi"("error in (no error)"=w496, "Force Delete (F)"=TRUE, "Item Ref in"=w497) -> ("error out"=w495:errorcluster)  [unwired: 7 in, 1 out]
                }
                n248 = Array Subset(array=w472, index=3) -> (w469:T11)  [unwired: 1 in]
                n249 = Array Subset(array=w467, index=3) -> (w465:T11)  [unwired: 1 in]
                n250 = Build Array (concatenate)(w469, w465) -> (w466:T11)
                n251 = for {
                  tunnel: w471 -> [w487]
                  shift-right: [w489] -> w474
                  shift-left: w470 -> [w486]
                  tunnel: w466 -> [w485] mode=indexing
                  n252 = Unbundle(w485) -> ("Channel Name"=w484:string)  [unwired: 2 out]
                  n253 = call-poly <vilib>:"NI VeriStand - Search for Item.vi"("error in"=w486, "Item Name"=w484, "Section Ref in"=w487) -> ("error out"=w488:errorcluster, "Item Refs"=w483:T2[])  [unwired: 5 in, 2 out]
                  n254 = for {
                    tunnel: w483 -> [w493] mode=indexing
                    shift-right: [w491] -> w489
                    shift-left: w488 -> [w492]
                    n255 = call <vilib>:"NI VeriStand - Remove Custom Device Item.vi"("error in (no error)"=w492, "Force Delete (F)"=TRUE, "Item Ref in"=w493) -> ("error out"=w491:errorcluster)  [unwired: 7 in, 1 out]
                  }
                }
                n256 = local write "Pullup Resistor Bank 0"(w475) -> ()
                n257 = local write "Pullup Resistor Bank 1"(w475) -> ()
              }
            }
          }
        }
        n258 = call <vilib>:"Simple Error Handler.vi"("error in (no error)"=w163) -> ("error out"=w162:errorcluster)  [unwired: 1 in, 7 out]
        n259 = call <vilib>:"Clear Errors.vi"("error in (no error)"=w162) -> ("error out"=w161:errorcluster)  [unwired: 1 in, 5 out]
      }
      n260 = Unregister For Events(event registration refnum=w155, error in=w154) -> (error out=w153:errorcluster)
    }
    frame Error {
      n261 = call <vilib>:"Simple Error Handler.vi"("error in (no error)"=w500) -> ("error out"=w499:errorcluster)  [unwired: 1 in, 7 out]
      n262 = call <vilib>:"Clear Errors.vi"("error in (no error)"=w499) -> ("error out"=w498:errorcluster)  [unwired: 1 in, 5 out]
    }
  }
  n263 = call <vilib>:"Clear Errors.vi"("error in (no error)"=w3) -> ()  [unwired: 5 in, 2 out]
  n264 = invoke class="VI" method="FP.Close"(error in=w25) -> (error out=w24:errorcluster)  [unwired: 2 in, 2 out]
  n265 = call <vilib>:"NI VeriStand - Signal When Ready for Shutdown.vi"("error in (no error)"=w24) -> ("error out"=→"error out":errorcluster)  [unwired: 10 out]
